vi "Read Binary Config.vi"(4 "Class Name is Included":bool, 6 "byte order (0:big-endian, network order)":T1(ring), 8 "error in (no error)":errorcluster, 10 "Binary":string, 11 "AbsFunc_One Term_I16 in":refnum<class "AbsFunc_One Term_I16.lvclass">) -> (0 "error out":errorcluster, 2 "Remaining":string, 3 "AbsFunc_One Term_I16 out":refnum<class "AbsFunc_One Term_I16.lvclass">)   [LabVIEW 2021, in "AbsFunc_One Term_I16.lvclass"]
uses:
  AbsFunc_One Term_I16.lvclass
  AbsFunc_One Term_I16.lvclass/AbsFunc_One Term_I16.ctl
  Abs_Types/I16 Integer/Abs_I16 Integer.lvclass
  C:/Users/Tim/Documents/GitHub/LV_Abstract/Source/Abs_Types/Type/Abs_Type.lvclass
  Abs_Types/Type/Abs_Type.lvclass
  C:/Users/Tim/Documents/GitHub/LV_Abstract/Source/Abs_Types/Integer/Abs_Integer.lvclass
  C:/Users/Tim/Documents/GitHub/LV_Abstract/Source/Abs_Types/Numeric/Abs_Numeric.lvclass
  C:/Users/Tim/Documents/GitHub/LV_Abstract/Source/Abs_Types/Value/Abs_Value.lvclass
  C:/Users/Tim/Documents/GitHub/LV_Abstract/Source/Abs_Types/I16 Integer/Abs_I16 Integer.lvclass
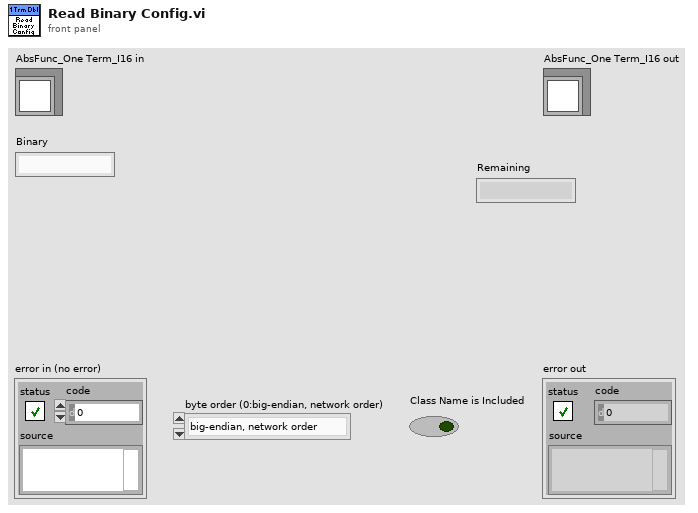
[diagram p1: front panel]
types:
  T1 = enum16{"big-endian, network order", "native, host order", "little-endian"}
  T2 = typedef "AbsFunc_One Term_I16.lvclass/Abstract Type.ctl" = refnum<class "Abs_I16 Integer.lvclass">
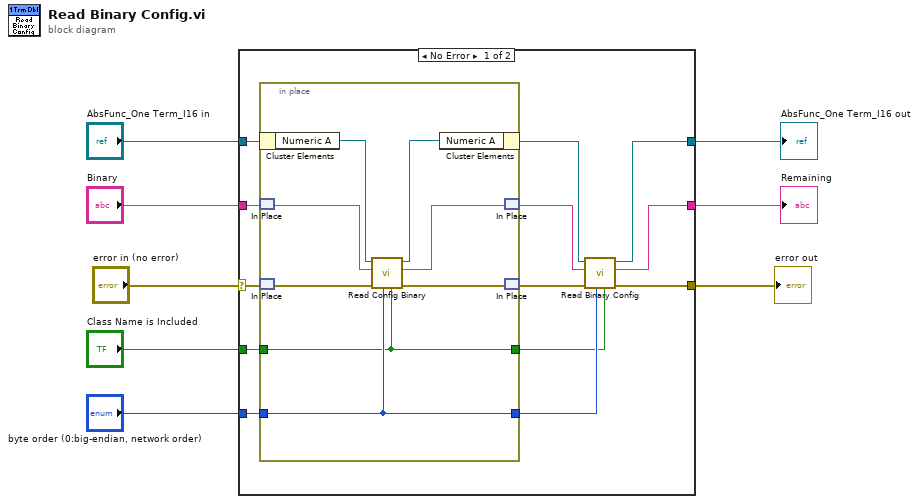
[diagram p0: block diagram]
diagram:
  n1 = case shown="No Error" "error in (no error)" {
    selector: "error in (no error)" -> [w20 w30]
    tunnel: "Binary" -> [w21 w31]
    tunnel: "AbsFunc_One Term_I16 in" -> [w19 w32]
    tunnel: [w15 w30] -> w8
    tunnel: [w14 w32] -> w1
    tunnel: "Class Name is Included" -> [w13 _]
    tunnel: "byte order (0:big-endian, network order)" -> [w12 _]
    tunnel: [w9 w31] -> w2
    frame No Error {
      n2 = in-place {
        in-place-border: w13 -> [w24]
        in-place-border: w12 -> [w25]
        in-place-border: [w25] -> w11
        in-place-border: [w24] -> w10
        n3 = in-place-cluster #1(w19) -> ("Numeric A"=w28:T2)
        n4 = in-place-match #2(w21) -> (w23:string)
        n5 = in-place-match #3(w20) -> (w29:errorcluster)
        n6 = call "Read Config Binary.vi"("Class Name is Included"=w24, "byte order (0:big-endian, network order)"=w25, "error in (no error)"=w29, "Binary"=w23, "Abs_Type in"=w28) -> ("error out"=w26:errorcluster, "Remaining"=w22:string, "Abs_Type in"=w27:T2)  [unwired: 4 in]
        n7 = in-place-cluster #1("Numeric A"=w27) -> (w16:refnum<class "AbsFunc_One Term_I16.lvclass">)
        n8 = in-place-match #2(w22) -> (w17:string)
        n9 = in-place-match #3(w26) -> (w18:errorcluster)
      }
      n10 = call-parent "Read Binary Config.vi"("Class Name is Included"=w10, "byte order (0:big-endian, network order)"=w11, "error in (no error)"=w18, "Binary"=w17, "Abs_Type in"=w16) -> ("error out"=w15:errorcluster, "Remaining"=w9:string, "Abs_Type out"=w14:refnum<class "AbsFunc_One Term_I16.lvclass">)  [unwired: 4 in]
    }
    frame Error {
    }
  }
  "error out" <- w8
  "AbsFunc_One Term_I16 out" <- w1
  "Remaining" <- w2
